vi "DAC_lines.vi"() -> ()   [LabVIEW 2010]
uses:
  <vilib>/Platform/TimedLoop/XDataNode/XDataNode.xnode
  <vilib>/Platform/TimedLoop/XDataNode/nitl_modes.ctl
  <vilib>/Platform/TimedLoop/XDataNode/XDNodeRunTimeDep.lvlib
  <vilib>/Platform/TimedLoop/XDataNode/wakeup.ctl
  <vilib>/Platform/TimedLoop/XDataNode/timing_clust.ctl
  <vilib>/eio/EIONode/EIONode.xnode
panel:
  in  "DIO 0-38":bool
  in  "DIO 0-36":bool
  in  "SYNC":bool
  in  "DIO 0-34":bool
  in  "DIO 0-32":bool
  in  "SCLK":bool
  in  "LDAC":bool
  in  "DIN":bool
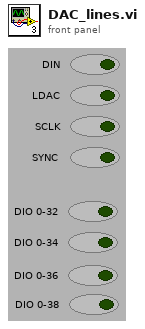
[diagram p1: front panel]
types:
  T1 = typedef "XDNodeRunTimeDep.lvlib/timing_clust.ctl" = cluster{"Expected End [f-1]":u64, "Actual End [f-1]":u64, "Finished Late? [f-1]":bool, "Expected End [i-1]":u64, "Actual End [i-1]":u64, "Finished Late? [i-1]":bool, "Expected Start [i]":u64, "Actual Start [i]":u64, "Expected Start [f]":u64, "Actual Start [f]":u64, "Source Name":string, "Structure Name":string, "Period":i64, "Deadline":i64, "Offset":i64, "Start":i64, "Priority":i32, "Timeout":i32, "Mode":T2, "Wakeup Reason":T3, "Error":errorcluster, "Source Type":string, "Secondary Source Type":string, "Global End Time":u64, "Global Start Time":u64, "Frame Duration":u64, "Iteration Duration":u64, "Assigned CPU":i32, "I/O Scan Engine Mode":u32}
  T2 = typedef "XDNodeRunTimeDep.lvlib/nitl_modes.ctl" = enum32{"No Change", "Process missed periods, maintain original phase", "Discard missed periods, maintain original phase", "Process missed periods, ignore original phase", "Discard missed periods, ignore original phase"}
  T3 = typedef "XDNodeRunTimeDep.lvlib/wakeup.ctl" = enum32{"Normal", "Aborted", "Asynchronous wakeup", "Timing source error", "Timed loop error", "Timeout"}
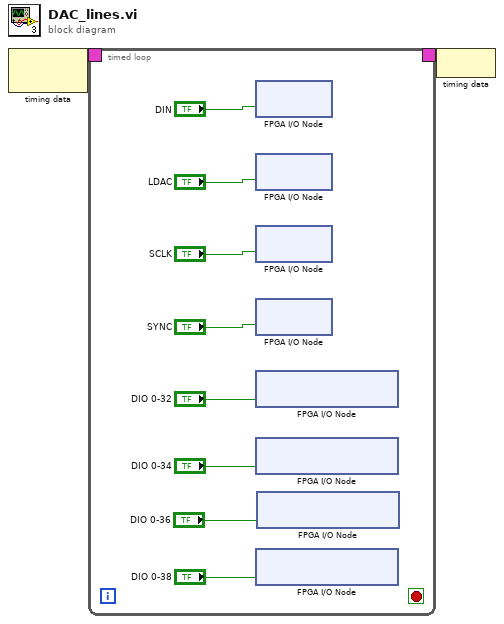
[diagram p0: block diagram]
diagram:
  n1 = node-c288() -> (w2:T1)  [unwired: 1 in]
  n2 = timed-loop {
    timing: w2 -> [_]
    timing-out: [_] -> w1
    stop <- _ stop-if-true
    n3 = xnode "FPGA I/O Node"("DIN"="DIN") -> ()  [unwired: 1 in, 1 out]
    n4 = xnode "FPGA I/O Node"("LDAC"="LDAC") -> ()  [unwired: 1 in, 1 out]
    n5 = xnode "FPGA I/O Node"("SCLK"="SCLK") -> ()  [unwired: 1 in, 1 out]
    n6 = xnode "FPGA I/O Node"("SYNC"="SYNC") -> ()  [unwired: 1 in, 1 out]
    n7 = xnode "FPGA I/O Node"("Connector0/DIO32"="DIO 0-32") -> ()  [unwired: 1 in, 1 out]
    n8 = xnode "FPGA I/O Node"("Connector0/DIO34"="DIO 0-34") -> ()  [unwired: 1 in, 1 out]
    n9 = xnode "FPGA I/O Node"("Connector0/DIO38"="DIO 0-38") -> ()  [unwired: 1 in, 1 out]
    n10 = xnode "FPGA I/O Node"("Connector0/DIO36"="DIO 0-36") -> ()  [unwired: 1 in, 1 out]
  }
  n11 = node-c288(w1) -> ()
